vi "Read Visible.vi"(8 "error in (no error)":errorcluster, 11 "GameEl in":refnum<class "GameEl.lvclass">) -> (0 "error out":errorcluster, 2 "Visible":bool, 3 "GameEl out":refnum<class "GameEl.lvclass">)   [LabVIEW 2021, in "GameEl.lvclass"]
uses:
  GameEl.lvclass
  GameEl.lvclass/GameEl.ctl
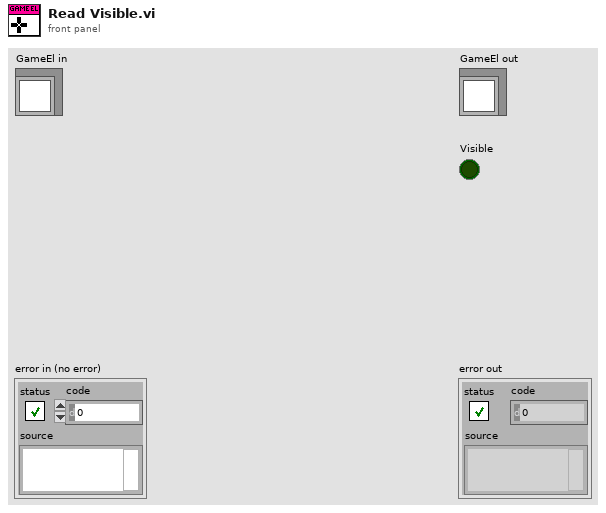
[diagram p1: front panel]
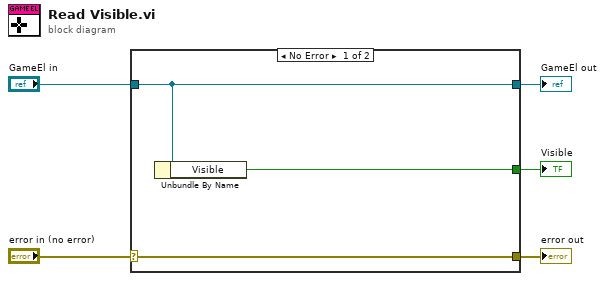
[diagram p0: block diagram]
diagram:
  n1 = case shown="No Error" "error in (no error)" {
    selector: "error in (no error)" -> [w8 w9]
    tunnel: [w8 w9] -> w4
    tunnel: [w7 w10] -> w2
    tunnel: "GameEl in" -> [w7 w10]
    tunnel: [w6 _] -> w1
    frame No Error {
      n2 = Unbundle By Name(w7) -> ("Visible"=w6:bool)
    }
    frame Error {
    }
  }
  "error out" <- w4
  "GameEl out" <- w2
  "Visible" <- w1
